vi "Get Hash Info.vi"(8 "error in (no error)":errorcluster, 11 "SHA-256 in":refnum<class "SHA-256.lvclass">) -> (0 "error out":errorcluster, 1 "Output Length (Bytes)":i32, 2 "Blocksize (Bytes)":i32, 3 "SHA-256 out":refnum<class "SHA-256.lvclass">)   [LabVIEW 2020, in "Crypto.lvlib" / "SHA-256.lvclass"]
uses:
  SHA-256.lvclass
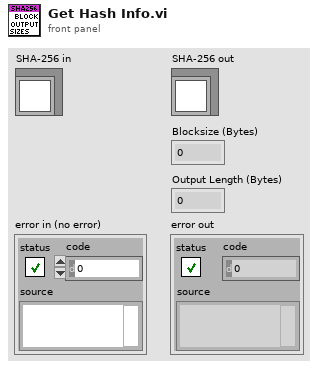
[diagram p1: front panel]
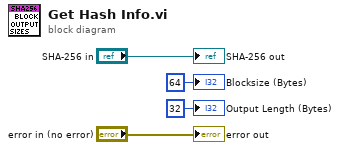
[diagram p0: block diagram]
diagram:
  "error out" <- "error in (no error)"
  "SHA-256 out" <- "SHA-256 in"
  "Blocksize (Bytes)" <- 64 ("Blocksize (Bytes)")
  "Output Length (Bytes)" <- 32 ("Output Length (Bytes)")
